vi "Set MCM Calculation Settings.vi"(7 "GUI Settings":T3, 8 "error in":errorcluster, 11 "MCM Calcualtion Settings":T1={"Repeats"=100, "Verbose"=TRUE, "Parallelization method"=enum."Single Core", "Processors"=1, "Temporary directory"=".", "Randomize"=TRUE} {"Processors" min=1 step=1; "Repeats" min=1 step=1}) -> (0 "error out":errorcluster)   [LabVIEW 2013]
uses:
  TD GUI Settings.ctl
  TD GUI Engine.ctl
  TD MCM Calculation Settings.ctl
  TD MCM Calculation Method.ctl
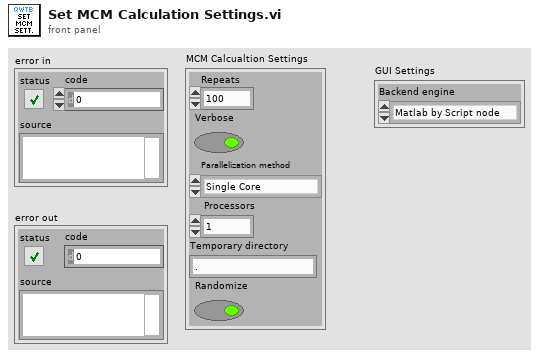
[diagram p1: front panel]
types:
  T1 = typedef "TD MCM Calculation Settings.ctl" = cluster{"Repeats":i32, "Verbose":bool, "Parallelization method":T2, "Processors":i32, "Temporary directory":string, "Randomize":bool}
  T2 = typedef "TD MCM Calculation Method.ctl" = enum16{"Single Core", "Multi Core", "Multi Station"}
  T3 = typedef "TD GUI Settings.ctl" = cluster{"Backend engine":T4}
  T4 = typedef "TD GUI Engine.ctl" = enum16{"Matlab by Script node", "GNU Octave by GOLPI"}
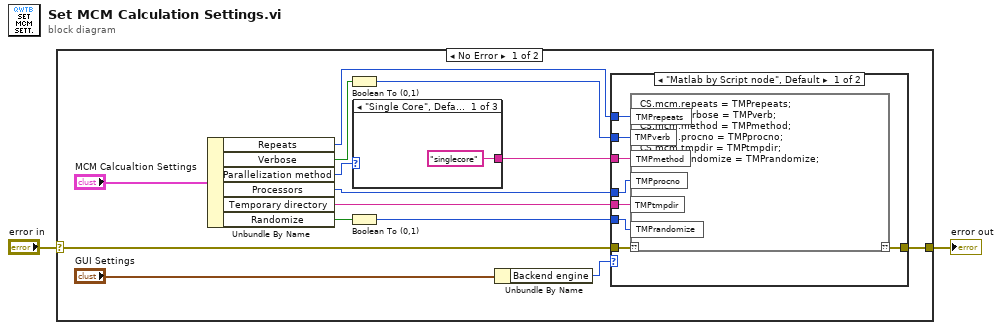
[diagram p0: block diagram]
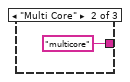
[diagram p3: hidden frame]
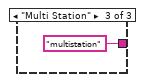
[diagram p4: hidden frame]
diagram:
  n1 = case shown="No Error" "error in" {
    selector: "error in" -> [w14 w29]
    tunnel: [w8 w29] -> w2
    frame No Error {
      n2 = Unbundle By Name("MCM Calcualtion Settings") -> ("Repeats"=w7:i32, "Verbose"=w13:bool, "Parallelization method"=w9:T2, "Processors"=w6:i32, "Temporary directory"=w5:string, "Randomize"=w4:bool)
      n3 = Boolean To (0,1)(Boolean=w13) -> (0, 1=w16:i16)
      n4 = Boolean To (0,1)(Boolean=w4) -> (0, 1=w3:i16)
      n5 = case shown="\"Single Core\", Default" w9 {
        tunnel: ["singlecore" ("String") "multicore" ("String") "multistation" ("String")] -> w15
        frame "Single Core", Default {
        }
        frame "Multi Core" {
        }
        frame "Multi Station" {
        }
      }
      n6 = Unbundle By Name("GUI Settings") -> ("Backend engine"=w12:T4)
      n7 = case shown="\"Matlab by Script node\", Default" w12 {
        tunnel: [w24 w25] -> w8
        tunnel: w16 -> [w23 _]
        tunnel: w15 -> [w22 _]
        tunnel: w14 -> [w21 w25]
        tunnel: w7 -> [w20 _]
        tunnel: w6 -> [w19 _]
        tunnel: w5 -> [w18 _]
        tunnel: w3 -> [w17 _]
        frame "Matlab by Script node", Default {
          n8 = script code="CS.mcm.repeats = TMPrepeats;\nCS.mcm.verbose = TMPverb;\nCS.mcm.method = TMPmethod;\nCS.mcm.procno = TMPprocno;\nCS.mcm.tmpdir = TMPtmpdir;\nCS.mcm.randomize = TMPrandomize;"("??"=w21, "TMPverb"=w23, "TMPmethod"=w22, "TMPrepeats"=w20, "TMPprocno"=w19, "TMPtmpdir"=w18, "TMPrandomize"=w17) -> ("??"=w24:errorcluster)
        }
        frame "GNU Octave by GOLPI" {
          # "#2DO"
        }
      }
    }
    frame Error {
    }
  }
  "error out" <- w2
